vi "cm2nm_update_fiducial_bynamematchr.vi"(1 "numbermatchedbyname":i32) -> (0 "Array":u32[](array[numeric]))   [LabVIEW 2011]
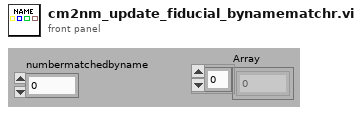
[diagram p1: front panel]
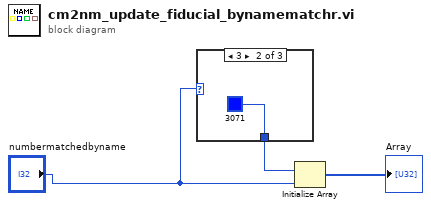
[diagram p0: block diagram]
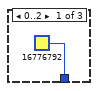
[diagram p2: hidden frame]
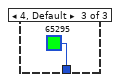
[diagram p3: hidden frame]
diagram:
  n1 = case shown="3" "numbermatchedbyname" {
    tunnel: [u32 16776792 u32 3071 u32 65295] -> w2
    frame 0..2 {
    }
    frame 3 {
    }
    frame 4, Default {
    }
  }
  n2 = Initialize Array(w2, "numbermatchedbyname") -> (→"Array":u32[])
